vi "Evaluate Digital Edge Trigger (Array).vi"(8 "error in (no error)":errorcluster, 10 "Trigger Data":dbl[](array[numeric]), 11 "Digital Edge Trigger in":refnum<class "Digital Edge Trigger.lvclass">) -> (0 "error out":errorcluster, 1 "Trigger indices":i32[](array[numeric]), 2 "Trigger":bool, 3 "Digital Edge Trigger out":refnum<class "Digital Edge Trigger.lvclass">)   [LabVIEW 2015, in "Waveform Data Logger Engine.lvlib" / "Digital Edge Trigger.lvclass"]
uses:
  Digital Edge Trigger.lvclass
  Digital Edge Trigger.lvclass/Digital Edge Trigger.ctl
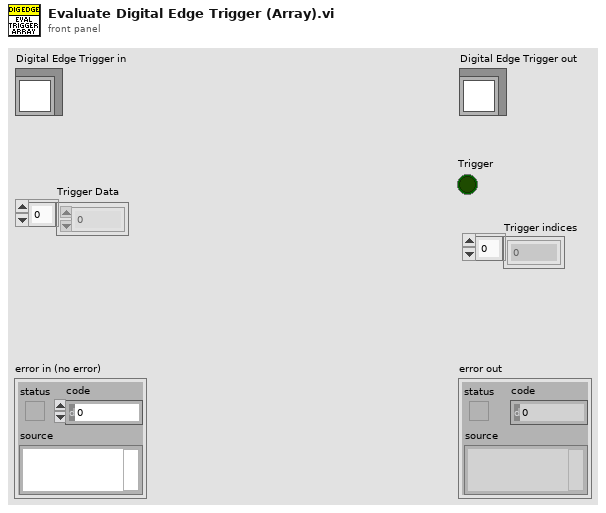
[diagram p1: front panel]
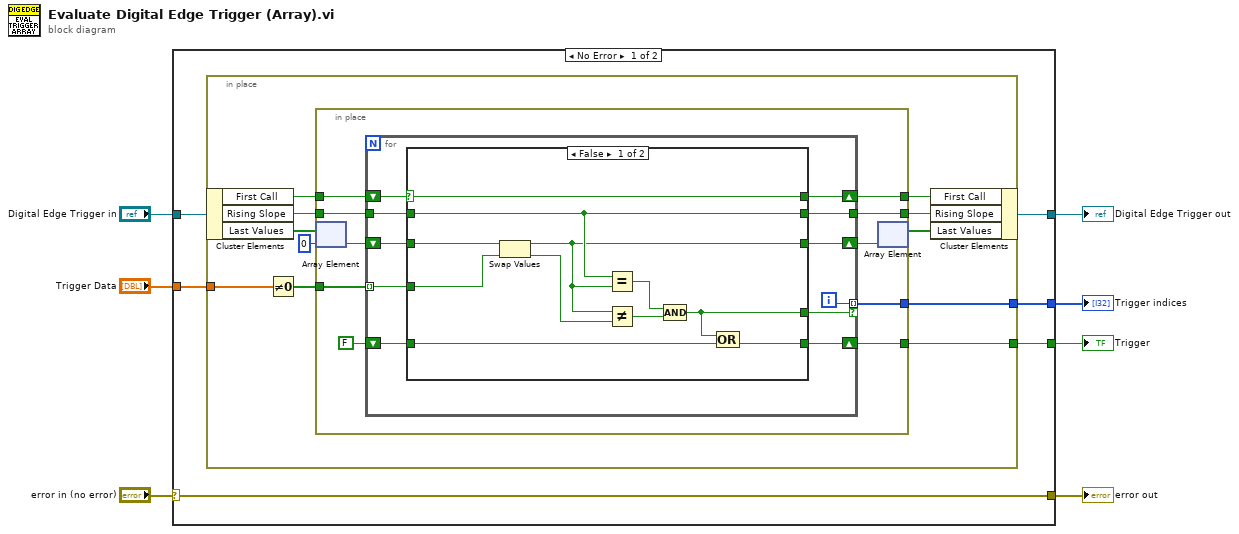
[diagram p0: block diagram]
diagram:
  n1 = case shown="No Error" "error in (no error)" {
    selector: "error in (no error)" -> [w9 w61]
    tunnel: "Digital Edge Trigger in" -> [w13 w60]
    tunnel: [w12 w60] -> w6
    tunnel: "Trigger Data" -> [w11 _]
    tunnel: [w10 _] -> w4
    tunnel: [w9 w61] -> w2
    tunnel: [w8 _] -> w1
    frame No Error {
      n2 = in-place {
        in-place-border: w11 -> [w19]
        in-place-border: [w22] -> w10
        in-place-border: [w14] -> w8
        n3 = in-place-cluster #1(w13) -> ("First Call"=w21:bool, "Rising Slope"=w24:bool, "Last Values"=w17:bool[])
        n4 = Not Equal To 0?(x=w19) -> (x != 0?=w18:bool[])
        n5 = in-place {
          in-place-border: w24 -> [w34]
          in-place-border: [w33] -> w23
          in-place-border: [w32] -> w22
          in-place-border: w21 -> [w31]
          in-place-border: [w30] -> w20
          in-place-border: w18 -> [w29]
          in-place-border: [w25] -> w14
          n6 = in-place-array #2(w17, 0) -> (w27:bool)
          n7 = for {
            tunnel: w34 -> [w45]
            tunnel: [w44] -> w33
            tunnel: w29 -> [w38] mode=indexing
            shift-right: [w41] -> w32
            shift-left: FALSE -> [w37]
            shift-right: [w39] -> w30
            shift-left: w31 -> [w40]
            shift-right: [w42] -> w26
            shift-left: w27 -> [w43]
            tunnel: [w36] -> w25 mode=indexing if=w35
            i -> [w36]
            n8 = case shown="False" w40 {
              selector: w40 -> [w52 _]
              tunnel: w45 -> [w54 w59]
              tunnel: [w54 w59] -> w44
              tunnel: w43 -> [w56 _]
              tunnel: [w53 w58] -> w42
              tunnel: [w55 w57] -> w41
              tunnel: [w52 _] -> w39
              tunnel: w38 -> [w51 w58]
              tunnel: w37 -> [w50 w57]
              tunnel: [w46 _] -> w35
              frame False {
                n9 = Swap Values(12:w56, 14:w51) -> (1:w53:bool, 3:w47:bool)  [unwired: 1 in]
                n10 = Equal?(x=w54, y=w53) -> (x = y?=w48:bool)
                n11 = Not Equal?(x=w53, y=w47) -> (x != y?=w49:bool)
                n12 = Compound Arithmetic op=AND(w48, w49) -> (w46:bool)
                n13 = Compound Arithmetic op=OR(w46, w50) -> (w55:bool)
              }
              frame True {
                # "Just latch the value on first call. The trigger takes at least two steps to trigger."
              }
            }
          }
          n14 = in-place-array #2(w26) -> (w15:bool[])  [unwired: 1 out]
        }
        n15 = in-place-cluster #1("First Call"=w20, "Rising Slope"=w23, "Last Values"=w15) -> (w12:refnum<class "Digital Edge Trigger.lvclass">)
      }
    }
    frame Error {
    }
  }
  "error out" <- w2
  "Digital Edge Trigger out" <- w6
  "Trigger" <- w4
  "Trigger indices" <- w1
